vi "MoindresCarres.vi"(8 "Ordre poly":u32, 9 "Y":sgl[](array[numeric]), 10 "X":sgl[](array[numeric]), 11 "Num pts":u32) -> (2 "Résidu":sgl, 3 "Meilleure poly":sgl[](array[numeric]))   [LabVIEW 2013]
panel:
  out "Points Ajustés":dbl[](array[numeric])
  in  "Points interpolation":u32=5 min=5 max=10000 step=1
  out "XY Graph":cluster{"X":sgl[], "Y":sgl[]}[](graph)
  in  "Calcul":bool
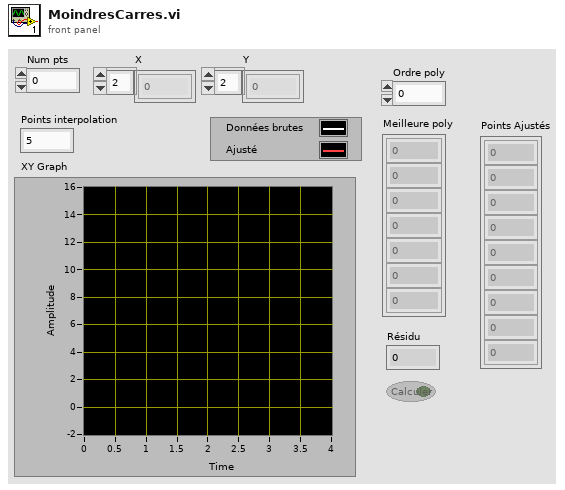
[diagram p1: front panel]
types:
  T1 = enum16{"Enabled", "Disabled", "Disabled and Grayed Out"}
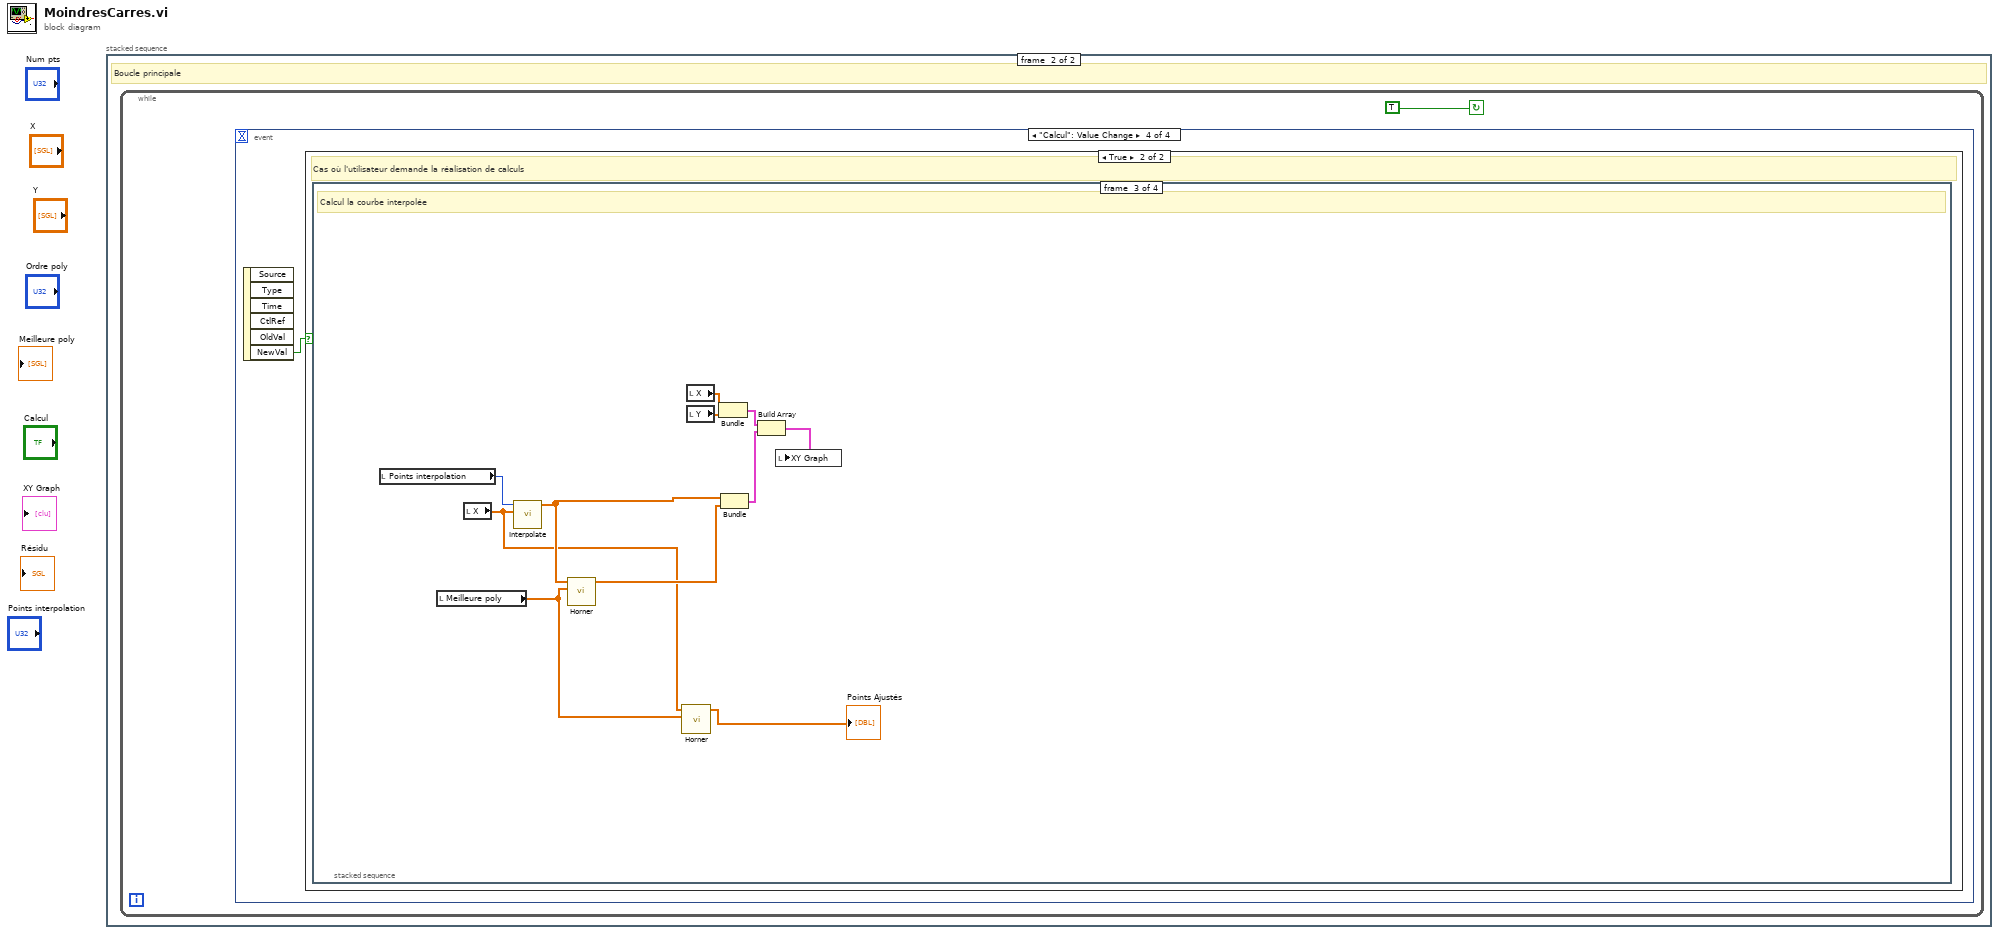
[diagram p0: block diagram]
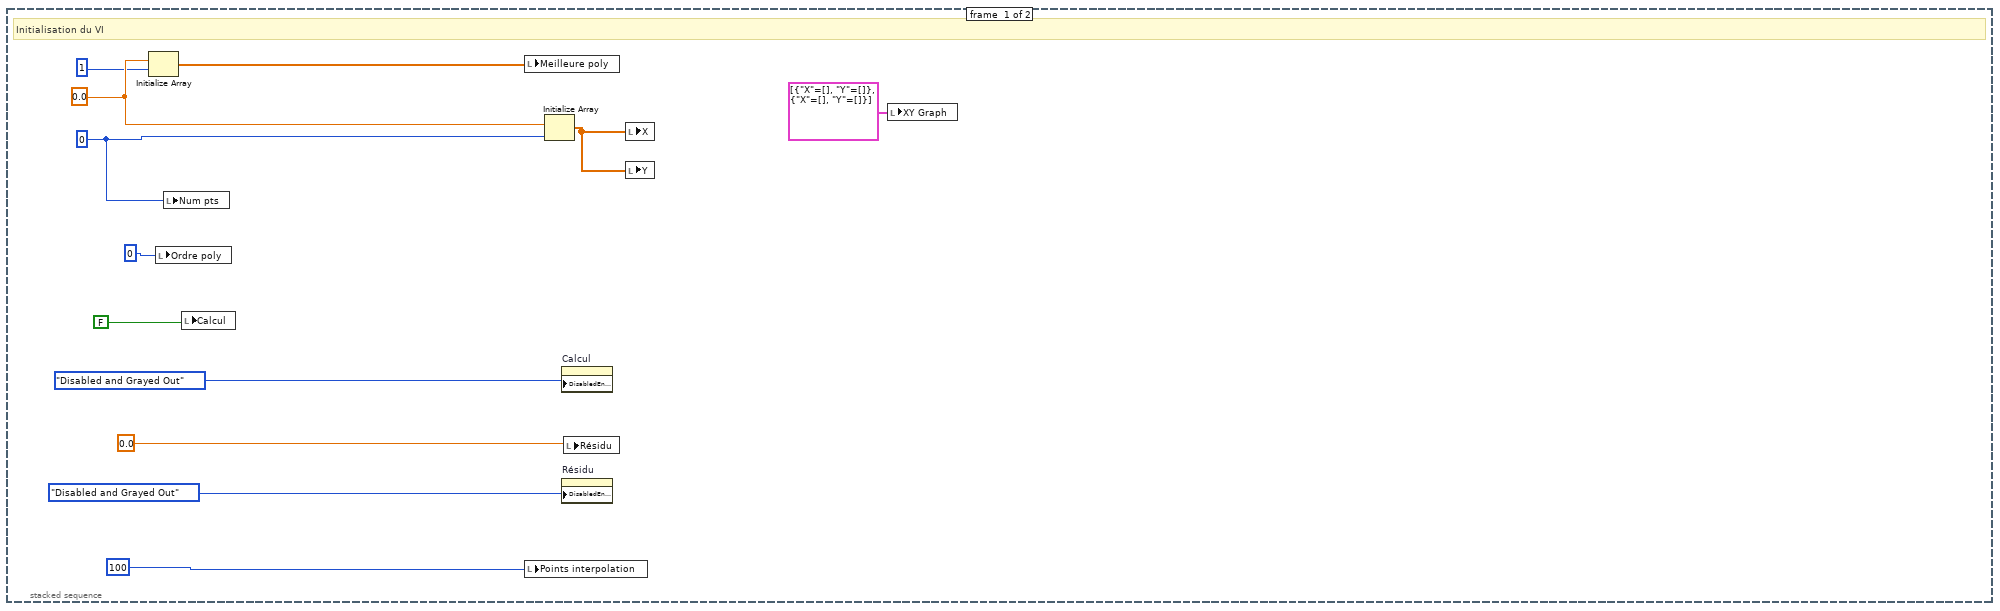
[diagram p2: hidden frame]
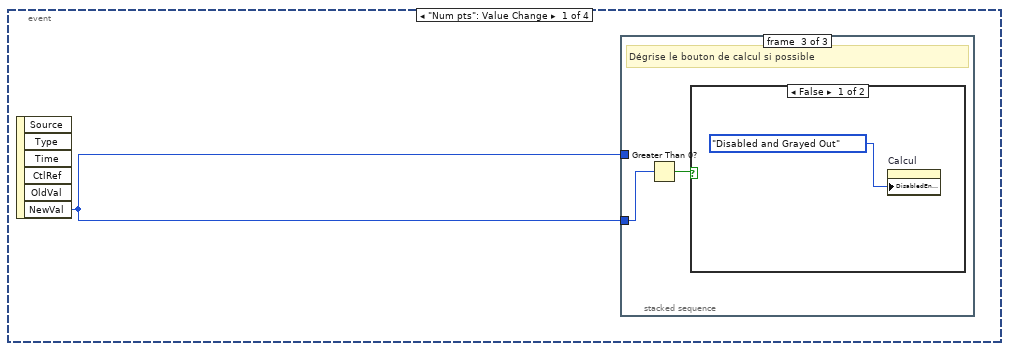
[diagram p3: hidden frame]
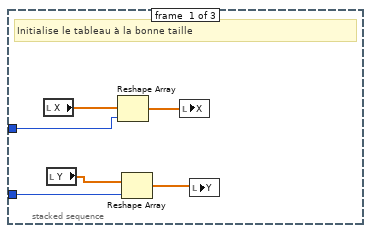
[diagram p4: hidden frame]
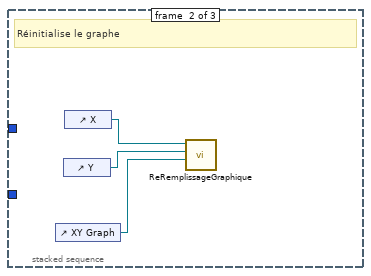
[diagram p5: hidden frame]
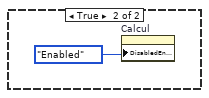
[diagram p6: hidden frame]
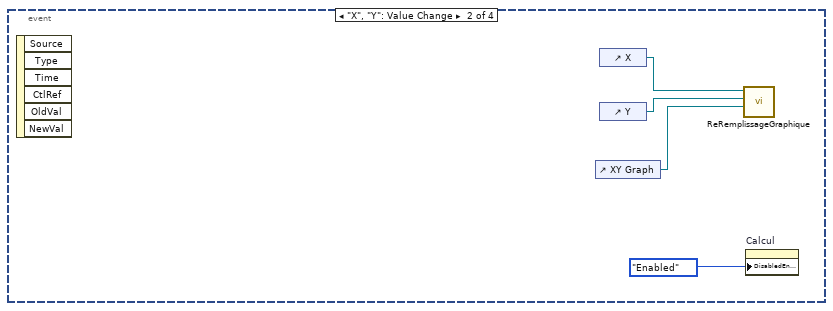
[diagram p7: hidden frame]
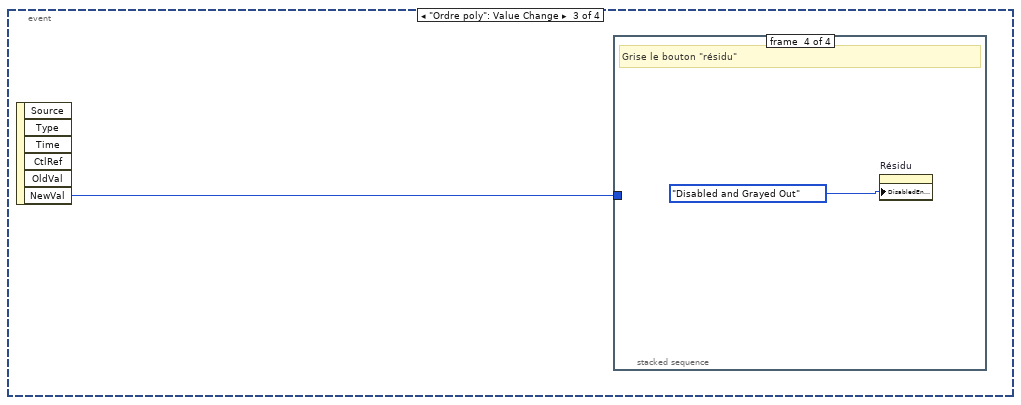
[diagram p8: hidden frame]
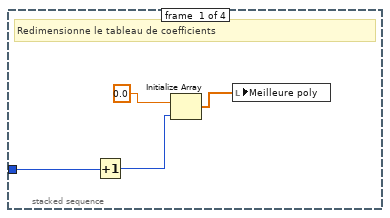
[diagram p9: hidden frame]
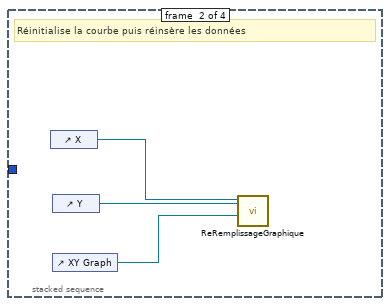
[diagram p10: hidden frame]
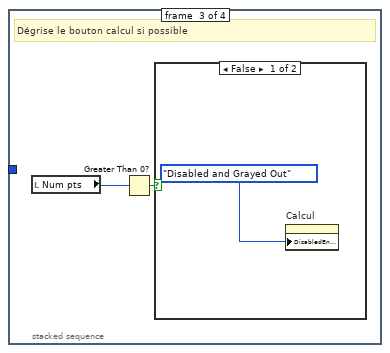
[diagram p11: hidden frame]
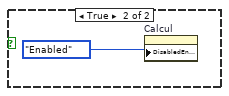
[diagram p12: hidden frame]
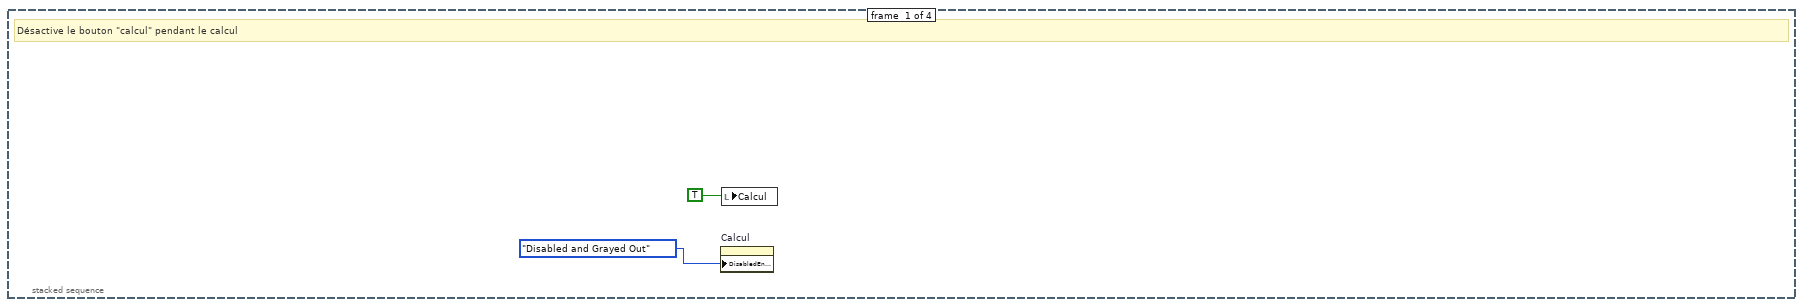
[diagram p14: hidden frame]
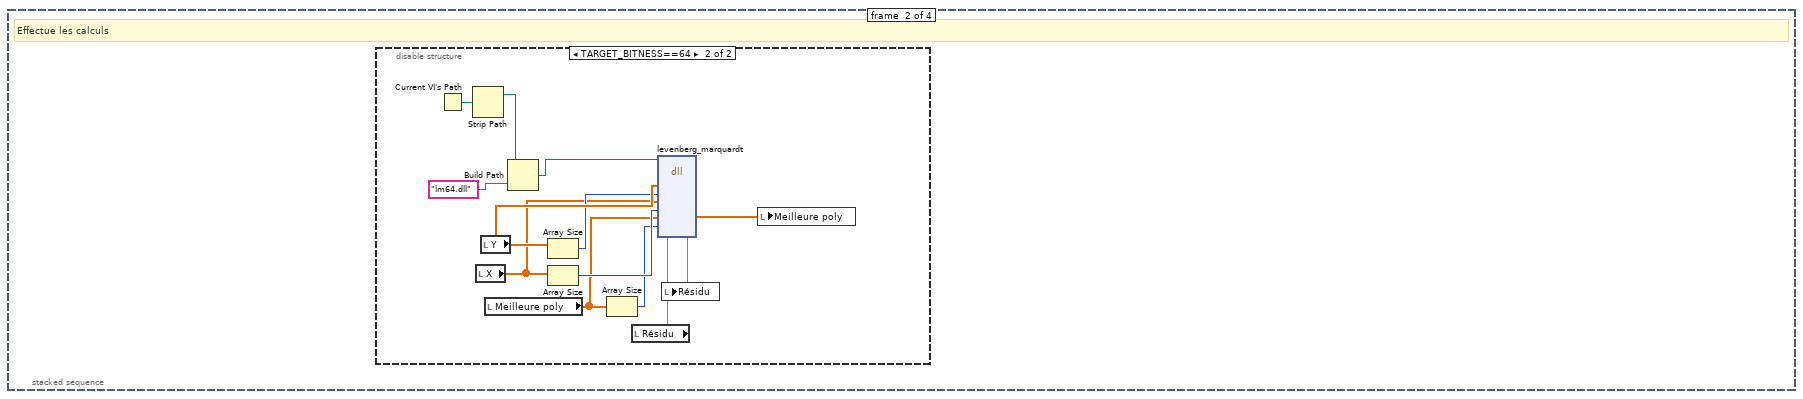
[diagram p15: hidden frame]
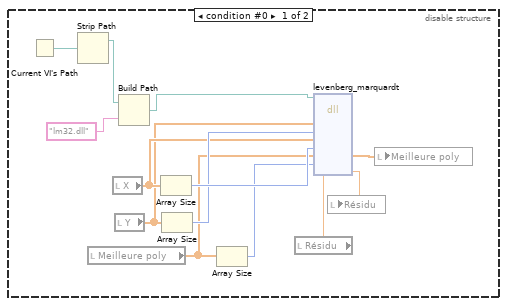
[diagram p16: hidden frame]
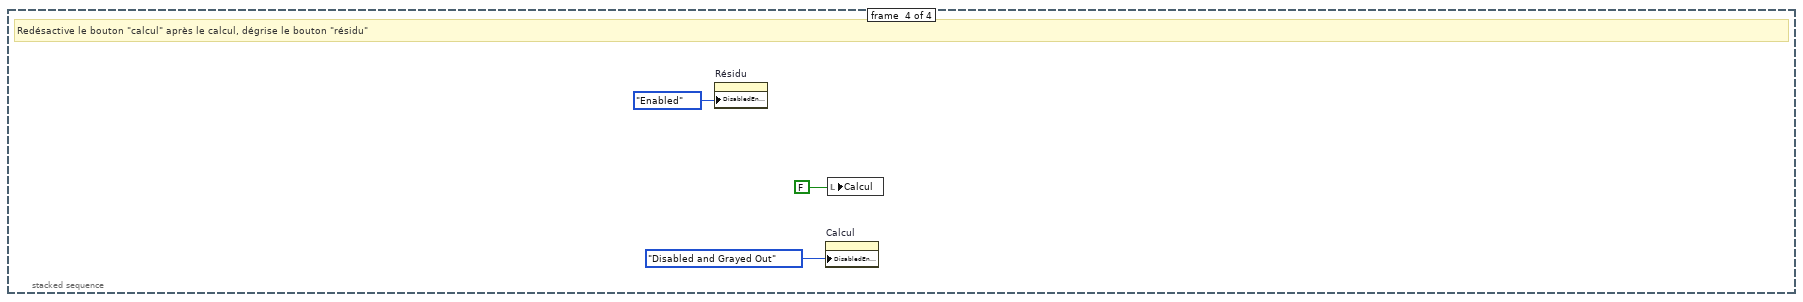
[diagram p17: hidden frame]
diagram:
  n1 = stacked-sequence {
    frame #0 {
      w8 = sgl 0.0
      w11 = 0
      # "Initialisation du VI"
      n2 = Initialize Array(w8, 1) -> (w10:sgl[])
      n3 = local write "Ordre poly"(0) -> ()
      n4 = local write "Num pts"(w11) -> ()
      n5 = local write "Calcul"(FALSE) -> ()
      n6 = local write "Meilleure poly"(w10) -> ()
      n7 = local write "Points interpolation"(100) -> ()
      n8 = Initialize Array(w8, w11) -> (w7:sgl[])
      n9 = property on="Calcul" class="Bool (strict)"("DisabledEnum"=T1."Disabled and Grayed Out") -> ()  [unwired: 2 in, 2 out]
      n10 = property on="Résidu" class="DigNum (strict)"("DisabledEnum"=T1."Disabled and Grayed Out") -> ()  [unwired: 2 in, 2 out]
      n11 = local write "Résidu"(0.0) -> ()
      n12 = local write "X"(w7) -> ()
      n13 = local write "Y"(w7) -> ()
      n14 = local write "XY Graph"(cluster{"X":sgl[], "Y":sgl[]}[] [{"X"=[], "Y"=[]}, {"X"=[], "Y"=[]}] ("XY Graph")) -> ()
    }
    frame #1 {
      # "Boucle principale"
      n15 = while {
        stop <- TRUE continue-if-true
        n16 = event shown="[3] \"Calcul\": Value Change" {
          selector: _ -> [_ _ _ _]
          dyn-events: _ -> [_ _ _ _]
          timeout: _ -> [_ _ _ _]
          event "Num pts": Value Change {
            n17 = event-data() -> ("NewVal"=w14:u32)  [unwired: 1 in, 5 out]
            n18 = stacked-sequence {
              tunnel: w14 -> [w18 _ w24]
              tunnel: w14 -> [w17 _ _]
              frame #0 {
                # "Initialise le tableau à la bonne taille"
                n19 = local read "X"() -> (w20:sgl[])
                n20 = local read "Y"() -> (w19:sgl[])
                n21 = Reshape Array(w20, w17) -> (w16:sgl[])
                n22 = Reshape Array(w19, w18) -> (w15:sgl[])
                n23 = local write "X"(w16) -> ()
                n24 = local write "Y"(w15) -> ()
              }
              frame #1 {
                # "Réinitialise le graphe"
                n25 = control-ref of="XY Graph"() -> (w21:refnum<vi>)
                n26 = control-ref of="Y"() -> (w22:refnum<vi>)
                n27 = control-ref of="X"() -> (w23:refnum<vi>)
                n28 = call "ReRemplissageGraphique.vi"("XY Graph ref"=w21, "Y arr ref"=w22, "X arr ref"=w23) -> ()  [unwired: 9 in]
              }
              frame #2 {
                # "Dégrise le bouton de calcul si possible"
                n29 = Greater Than 0?(x=w24) -> (x > 0?=w25:bool)
                n30 = case shown="False" w25 {
                  frame False {
                    n31 = property on="Calcul" class="Bool (strict)"("DisabledEnum"=T1."Disabled and Grayed Out") -> ()  [unwired: 2 in, 2 out]
                  }
                  frame True {
                    n32 = property on="Calcul" class="Bool (strict)"("DisabledEnum"=T1."Enabled") -> ()  [unwired: 2 in, 2 out]
                  }
                }
              }
            }
          }
          event "X", "Y": Value Change {
            n33 = event-data() -> ()  [unwired: 1 in, 6 out]
            n34 = control-ref of="XY Graph"() -> (w31:refnum<vi>)
            n35 = control-ref of="X"() -> (w29:refnum<vi>)
            n36 = control-ref of="Y"() -> (w30:refnum<vi>)
            n37 = call "ReRemplissageGraphique.vi"("XY Graph ref"=w31, "Y arr ref"=w30, "X arr ref"=w29) -> ()  [unwired: 9 in]
            n38 = property on="Calcul" class="Bool (strict)"("DisabledEnum"=T1."Enabled") -> ()  [unwired: 2 in, 2 out]
          }
          event "Ordre poly": Value Change {
            n39 = event-data() -> ("NewVal"=w32:u32)  [unwired: 1 in, 5 out]
            n40 = stacked-sequence {
              tunnel: w32 -> [w36 _ _ _]
              frame #0 {
                # "Redimensionne le tableau de coefficients"
                n41 = Increment(x=w36) -> (x+1=w34:u32)
                n42 = Initialize Array(0.0, w34) -> (w33:dbl[])
                n43 = local write "Meilleure poly"(w33) -> ()
              }
              frame #1 {
                # "Réinitialise la courbe puis réinsère les données"
                n44 = control-ref of="X"() -> (w39:refnum<vi>)
                n45 = control-ref of="Y"() -> (w38:refnum<vi>)
                n46 = control-ref of="XY Graph"() -> (w37:refnum<vi>)
                n47 = call "ReRemplissageGraphique.vi"("XY Graph ref"=w37, "Y arr ref"=w38, "X arr ref"=w39) -> ()  [unwired: 9 in]
              }
              frame #2 {
                # "Dégrise le bouton calcul si possible"
                n48 = local read "Num pts"() -> (w40:u32)
                n49 = Greater Than 0?(x=w40) -> (x > 0?=w41:bool)
                n50 = case shown="False" w41 {
                  frame False {
                    n51 = property on="Calcul" class="Bool (strict)"("DisabledEnum"=T1."Disabled and Grayed Out") -> ()  [unwired: 2 in, 2 out]
                  }
                  frame True {
                    n52 = property on="Calcul" class="Bool (strict)"("DisabledEnum"=T1."Enabled") -> ()  [unwired: 2 in, 2 out]
                  }
                }
              }
              frame #3 {
                # "Grise le bouton \"résidu\""
                n53 = property on="Résidu" class="DigNum (strict)"("DisabledEnum"=T1."Disabled and Grayed Out") -> ()  [unwired: 2 in, 2 out]
              }
            }
          }
          event "Calcul": Value Change {
            n54 = event-data() -> ("NewVal"=w45:bool)  [unwired: 1 in, 5 out]
            n55 = case shown="True" w45 {
              frame False {
              }
              frame True {
                # "Cas où l'utilisateur demande la réalisation de calculs"
                n56 = stacked-sequence {
                  frame #0 {
                    # "Désactive le bouton \"calcul\" pendant le calcul"
                    n57 = property on="Calcul" class="Bool (strict)"("DisabledEnum"=T1."Disabled and Grayed Out") -> ()  [unwired: 2 in, 2 out]
                    n58 = local write "Calcul"(TRUE) -> ()
                  }
                  frame #1 {
                    # "Effectue les calculs"
                    n59 = disable-structure shown="TARGET_BITNESS==64" {
                      frame condition #0 {
                        n60 = Current VI's Path() -> (path=w48:path)
                        n61 = Strip Path(path=w48) -> (stripped path=w49:path)  [unwired: 1 out]
                        n62 = local read "Meilleure poly"() -> (w51:sgl[])
                        n63 = local read "X"() -> (w56:sgl[])
                        n64 = local read "Y"() -> (w55:sgl[])
                        n65 = Build Path(base path=w49, name or relative path="lm32.dll") -> (appended path=w59:path)
                        n66 = Array Size(array=w56) -> (size(s)=w58:i32)
                        n67 = Array Size(array=w55) -> (size(s)=w57:i32)
                        n68 = Array Size(array=w51) -> (size(s)=w50:i32)
                        n69 = local read "Résidu"() -> (w54:sgl)
                        n70 = dll-call lib="?" fn="levenberg_marquardt"(path in=w59, "yobs"=w55, "yobsLength"=w57, "xobs"=w56, "xobsLength"=w58, "polyptr"=w51, "numCoeffs"=w50, "e"=w54) -> ("polyptr"=w52:sgl[], "e"=w53:sgl)  [unwired: 8 in, 2 out]
                        n71 = local write "Résidu"(w53) -> ()
                        n72 = local write "Meilleure poly"(w52) -> ()
                      }
                      frame condition #1 (active) {
                        n73 = Current VI's Path() -> (path=w63:path)
                        n74 = Strip Path(path=w63) -> (stripped path=w62:path)  [unwired: 1 out]
                        n75 = local read "X"() -> (w70:sgl[])
                        n76 = local read "Y"() -> (w72:sgl[])
                        n77 = local read "Meilleure poly"() -> (w67:sgl[])
                        n78 = Build Path(base path=w62, name or relative path="lm64.dll") -> (appended path=w61:path)
                        n79 = Array Size(array=w72) -> (size(s)=w71:i32)
                        n80 = Array Size(array=w70) -> (size(s)=w69:i32)
                        n81 = Array Size(array=w67) -> (size(s)=w68:i32)
                        n82 = local read "Résidu"() -> (w66:sgl)
                        n83 = dll-call lib="?" fn="levenberg_marquardt"(path in=w61, "yobs"=w72, "yobsLength"=w71, "xobs"=w70, "xobsLength"=w69, "polyptr"=w67, "numCoeffs"=w68, "e"=w66) -> ("polyptr"=w65:sgl[], "e"=w64:sgl)  [unwired: 8 in, 2 out]
                        n84 = local write "Résidu"(w64) -> ()
                        n85 = local write "Meilleure poly"(w65) -> ()
                      }
                    }
                  }
                  frame #2 {
                    # "Calcul la courbe interpolée"
                    n86 = local read "Points interpolation"() -> (w79:u32)
                    n87 = local read "Meilleure poly"() -> (w76:sgl[])
                    n88 = local read "X"() -> (w75:sgl[])
                    n89 = call "Interpolate.vi"("X"=w75, "Points interpolation"=w79) -> ("Array"=w77:sgl[])  [unwired: 9 in]
                    n90 = call "Horner.vi"("Meilleure poly"=w76, "X"=w77) -> ("Y"=w78:sgl[])  [unwired: 9 in]
                    n91 = call "Horner.vi"("Meilleure poly"=w76, "X"=w75) -> ("Y"=→"Points Ajustés":sgl[])  [unwired: 9 in]
                    n92 = local read "X"() -> (w83:sgl[])
                    n93 = local read "Y"() -> (w84:sgl[])
                    n94 = Bundle("X"=w83, "Y"=w84) -> (w82:cluster{"X":sgl[], "Y":sgl[]})  [unwired: 1 in]
                    n95 = Bundle("Array"=w77, "Y"=w78) -> (w81:cluster{"Array":sgl[], "Y":sgl[]})  [unwired: 1 in]
                    n96 = Build Array(w82, w81) -> (w80:cluster{"Array":sgl[], "Y":sgl[]}[])
                    n97 = local write "XY Graph"(w80) -> ()
                  }
                  frame #3 {
                    # "Redésactive le bouton \"calcul\" après le calcul, dégrise le bouton \"résidu\""
                    n98 = property on="Résidu" class="DigNum (strict)"("DisabledEnum"=T1."Enabled") -> ()  [unwired: 2 in, 2 out]
                    n99 = property on="Calcul" class="Bool (strict)"("DisabledEnum"=T1."Disabled and Grayed Out") -> ()  [unwired: 2 in, 2 out]
                    n100 = local write "Calcul"(FALSE) -> ()
                  }
                }
              }
            }
          }
        }
      }
    }
  }
